vi "SSL_Connect_With_Keys.vi"(8 "error in (no error)":errorcluster, 9 "cert path":T1={"client cert file"=path "", "client key file"=path ""}, 10 "SSL_Connection":T2, 11 "login":T3={"server IP"="", "server port"=0, "local port (0 = auto)"=0, "timeout ms (1000)"=1000}) -> (0 "error out":errorcluster, 2 "SSL_Connection":T2)   [LabVIEW 2018, in "AWS_IoT.lvlib"]
doc: "Make the SSL connection.\nMIT License\n\nCopyright (c) 2016 Indie-Energy\n\nPermission is hereby granted, free of charge, to any person obtaining a copy\nof this software and associated documentation files (the \"Software\"), to deal\nin the Software without restriction, including without limitation the rights\nto use, copy, modify, merge, publish, distribute, sublicense, and/or sell\ncopies of the Software, and to permit persons to whom the Software is\nfurnished to do so, subject to the following conditions:\n\nThe above copyright notice and this permission notice shall be included in all\ncopies or substantial portions of the Software.\n\nTHE SOFTWARE IS PROVIDED \"AS IS\", WITHOUT WARRANTY OF ANY KIND, EXPRESS OR\nIMPLIED, INCLUDING BUT NOT LIMITED TO THE WARRANTIES OF MERCHANTABILITY,\nFITNESS FOR A PARTICULAR PURPOSE AND NONINFRINGEMENT. IN NO EVENT SHALL THE\nAUTHORS OR COPYRIGHT HOLDERS BE LIABLE FOR ANY CLAIM, DAMAGES OR OTHER\nLIABILITY, WHETHER IN AN ACTION OF CONTRACT, TORT OR OTHERWISE, ARISING FROM,\nOUT OF OR IN CONNECTION WITH THE SOFTWARE OR THE USE OR OTHER DEALINGS IN THE\nSOFTWARE."
uses:
  AWS_IoT.lvlib
  Controls/SSL_login.ctl
  Controls/SSL_Connection.ctl
  Controls/certs.ctl
panel:
  out "Numeric":i32
  out "return type 2":i32
  out "return type":i32
  out "connection status":i32
  out "retCode":i32
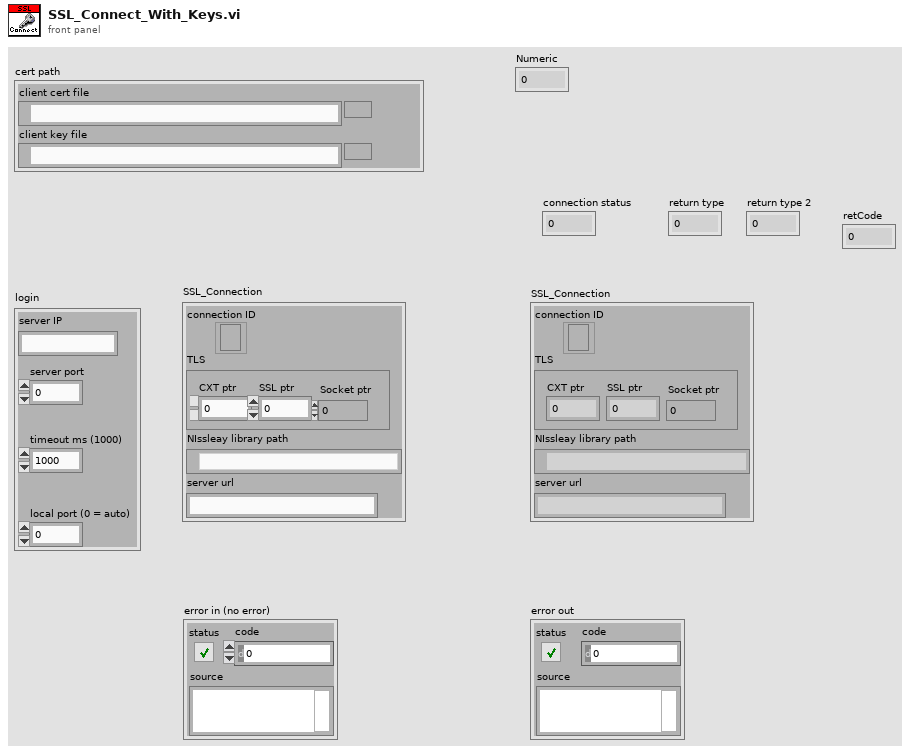
[diagram p1: front panel]
types:
  T1 = typedef "AWS_IoT.lvlib/certs.ctl" = cluster{"client cert file":path, "client key file":path}
  T2 = typedef "AWS_IoT.lvlib/SSL_Connection.ctl" = cluster{"connection ID":refnum<k5>, "TLS":cluster{"CXT ptr":i32, "SSL ptr":i32, "Socket ptr":i32}, "NIssleay library path":path, "server url":string}
  T3 = typedef "AWS_IoT.lvlib/SSL_login.ctl" = cluster{"server IP":string, "server port":u16, "local port (0 = auto)":u16, "timeout ms (1000)":i32}
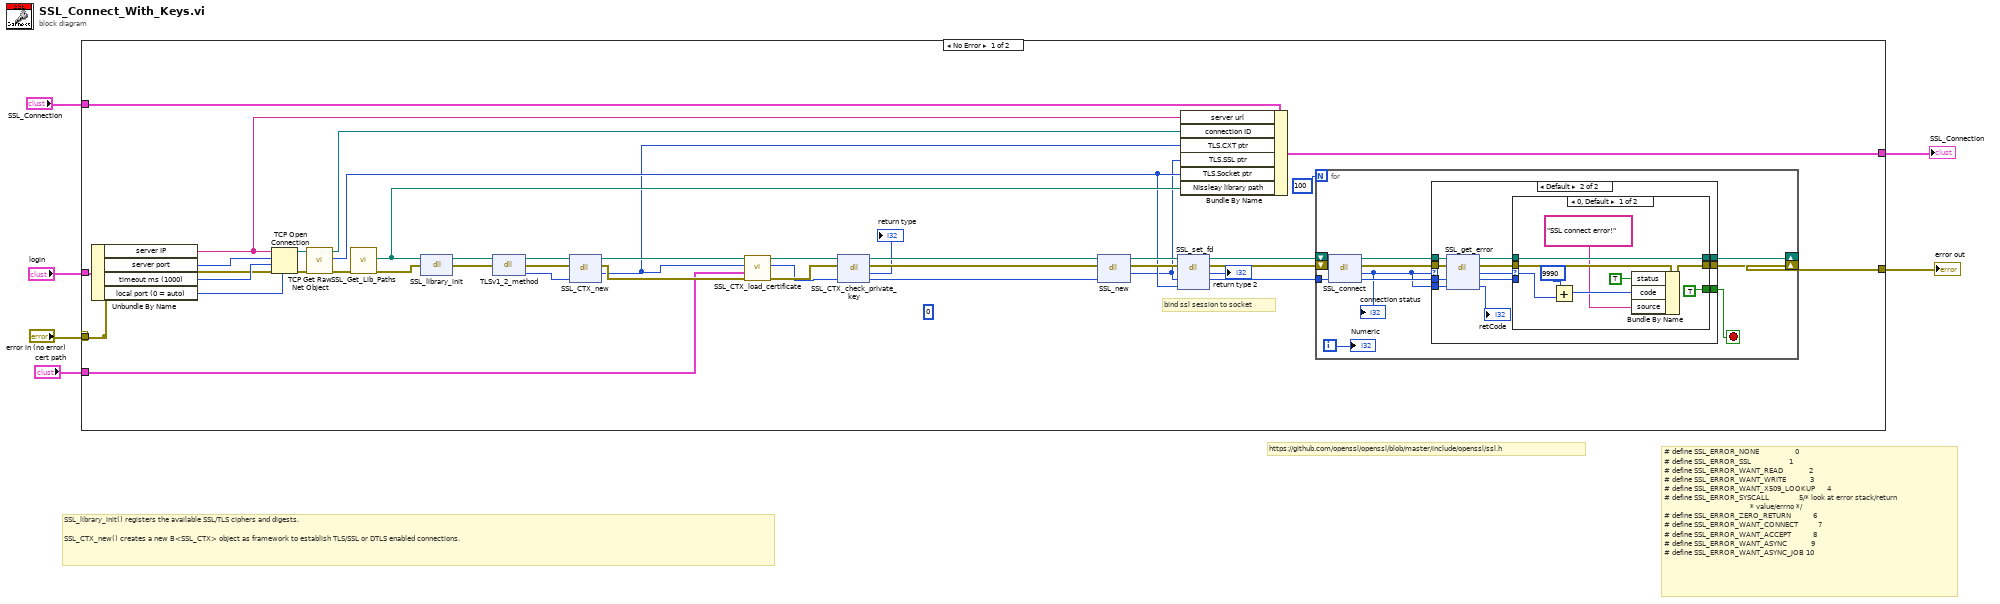
[diagram p0: block diagram]
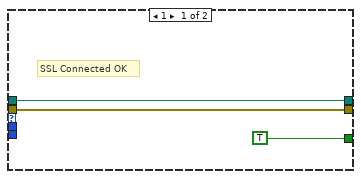
[diagram p2: hidden frame]
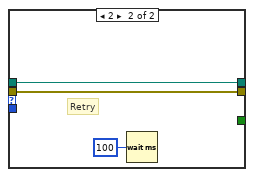
[diagram p3: hidden frame]
diagram:
  # "https://github.com/openssl/openssl/blob/master/include/openssl/ssl.h"
  # "# define SSL_ERROR_NONE                  0\n# define SSL_ERROR_SSL                   1\n# define SSL_ERROR_WANT_READ             2\n# define SSL_ERROR_WANT_WRITE            3\n# define SSL_ERROR_WANT_X509_LOOKUP      4\n# define SSL_ERROR_SYSCALL               5/* look at error stack/return\n                                           * value/errno */\n# define SSL_ERROR_ZERO_RETURN           6\n# define SSL_ERROR_WANT_CONNECT          7\n# define SSL_ERROR_WANT_ACCEPT           8\n# define SSL_ERROR_WANT_ASYNC            9\n# define SSL_ERROR_WANT_ASYNC_JOB 10"
  # "SSL_library_init() registers the available SSL/TLS ciphers and digests.\n\nSSL_CTX_new() creates a new B<SSL_CTX> object as framework to establish TLS/SSL or DTLS enabled connections."
  n1 = case shown="No Error" "error in (no error)" {
    selector: "error in (no error)" -> [w7 w85]
    tunnel: "login" -> [w41 _]
    tunnel: "SSL_Connection" -> [w40 w86]
    tunnel: [w27 w86] -> w4
    tunnel: [w7 _] -> _
    tunnel: [w8 w85] -> w3
    tunnel: "cert path" -> [w14 _]
    frame No Error {
      (unwired) 0 ("verify_callback")
      # "bind ssl session to socket"
      n2 = Unbundle By Name(w41) -> ("server IP"=w24:string, "server port"=w44:u16, "timeout ms (1000)"=w43:i32, "local port (0 = auto)"=w42:u16)
      n3 = TCP Open Connection(address=w24, remote port or service name=w44, timeout ms (60000)=w43, local port=w42, error in (no error)=w7) -> (connection ID=w46:refnum<k5>, error out=w45:errorcluster)
      n4 = call <vilib>:"TCP Get Raw Net Object.vi"("error in (no error)"=w45, "connection ID"=w46) -> ("error out"=w31:errorcluster, "raw net object"=w28:u64, "connection ID out"=w39:refnum<k5>)  [unwired: 7 in]
      n5 = call "SSL_Get_Lib_Paths.vi"("error in (no error)"=w31) -> ("error out"=w29:errorcluster, "NIssleay"=w30:path)  [unwired: 9 in]
      n6 = dll-call lib="NIssleay32.*" fn="SSL_library_init"(path in=w30, error in=w29) -> (path out=w37:path, error out=w32:errorcluster)  [unwired: 2 in]
      n7 = dll-call lib="NIssleay32.*" fn="TLSv1_2_method"(path in=w37, error in=w32) -> (path out=w38:path, error out=w33:errorcluster, "return type"=w34:i32)  [unwired: 1 in]
      n8 = dll-call lib="NIssleay32.*" fn="SSL_CTX_new"(path in=w38, error in=w33, "ClientMethod"=w34) -> (path out=w18:path, error out=w16:errorcluster, "return type"=w15:i32)  [unwired: 2 in]
      n9 = call "SSL_CTX_load_certificate.vi"("error in (no error)"=w16, "cert path"=w14, "CTX"=w15, "path in"=w18) -> ("error out"=w13:errorcluster, "CTX"=w12:i32, "path out"=w17:path)  [unwired: 5 in]
      n10 = dll-call lib="NIssleay32.*" fn="SSL_CTX_check_private_key"(path in=w17, error in=w13, "CTX"=w12) -> (path out=w22:path, error out=w21:errorcluster, "return type"=→"return type":i32, "CTX"=w20:i32)  [unwired: 1 in]
      n11 = dll-call lib="NIssleay32.*" fn="SSL_new"(path in=w22, error in=w21, "Context"=w20) -> (path out=w35:path, error out=w36:errorcluster, "return type"=w9:i32)  [unwired: 2 in]
      n12 = dll-call lib="NIssleay32.*" fn="SSL_set_fd"(path in=w35, error in=w36, "SSL"=w9, "Socket"=w28) -> (path out=w26:path, error out=w25:errorcluster, "return type"=→"return type 2":i32, "SSL"=w23:i32)  [unwired: 2 in]
      n13 = Bundle By Name(cluster=w40, "server url"=w24, "connection ID"=w39, "TLS.CXT ptr"=w15, "TLS.SSL ptr"=w9, "TLS.Socket ptr"=w28, "NIssleay library path"=w30) -> (w27:T2)
      n14 = for {
        N: 100 -> [_]
        tunnel: w23 -> [w54]
        shift-right: [w55] -> _
        shift-left: w26 -> [w57]
        shift-right: [w53] -> w8
        shift-left: w25 -> [w56]
        i -> [w48]
        stop <- w47 stop-if-true
        n15 = dll-call lib="NIssleay32.*" fn="SSL_connect"(path in=w57, error in=w56, "SSL"=w54) -> (path out=w52:path, error out=w51:errorcluster, "return type"=w49:i32, "SSL"=w50:i32)  [unwired: 1 in]
        "connection status" <- w49
        n16 = case shown="Default" w49 {
          tunnel: w49 -> [_ w72]
          tunnel: w52 -> [w60 w71]
          tunnel: w51 -> [w59 w70]
          tunnel: [w59 w66] -> w53
          tunnel: [TRUE w64] -> w47
          tunnel: w50 -> [_ w63]
          tunnel: [w60 w67] -> w55
          frame 1 {
            # "SSL Connected OK"
          }
          frame Default {
            n17 = dll-call lib="NIssleay32.*" fn="SSL_get_error"(path in=w71, error in=w70, "SSL"=w63, "retCode"=w72) -> (path out=w68:path, error out=w69:errorcluster, "return type"=w65:i32, "SSL"=w62:i32, "retCode"=→"retCode":i32)  [unwired: 1 in]
            n18 = case shown="0, Default" w65 {
              selector: w65 -> [w79 _]
              tunnel: w69 -> [w77 w82]
              tunnel: w68 -> [w81 w83]
              tunnel: [w81 w83] -> w67
              tunnel: [w76 w82] -> w66
              tunnel: [TRUE _] -> w64
              tunnel: w62 -> [_ _]
              frame 0, Default {
                n19 = Add(x=9990, y=w79) -> (x+y=w74:i32)
                n20 = Bundle By Name(cluster=w77, "status"=TRUE, "code"=w74, "source"="SSL connect error!" ("error message (\"\")")) -> (w76:errorcluster)
              }
              frame 2 {
                # "Retry"
                n21 = Wait (ms)(milliseconds to wait=u32 100) -> ()  [unwired: 1 out]
              }
            }
          }
        }
        "Numeric" <- w48
      }
    }
    frame Error {
    }
  }
  "SSL_Connection" <- w4
  "error out" <- w3
